vi "Process.vi"(9 "process sync":refnum<notifier>, 10 "TopLevel":refnum<class "TopLevel.lvclass">, 11 "Database in":refnum<class "Database.lvclass">) -> ()   [LabVIEW 2022 SP3, in "Database.lvclass"]
doc: "Developed by Kevin Thompson\nkevin@thompsonengineering.net\n\nCopyright 2018\nThompson Engineering, LLC"
uses:
  Database.lvclass
  DataTypes/Read Data--cluster.ctl
  TopLevel/TopLevel.lvclass
  DataTypes/Process - AppData--cluster.ctl
  DataTypes/Settings--cluster.ctl
  DataTypes/Dependency--cluster.ctl
  DataTypes/Public Events--cluster.ctl
  Common/Controls/TD Async CmdMsg EventData--cluster.ctl
  Common/Controls/TD Sync API Event Data.ctl
  Common/Controls/APIReturnCluster--Cluster.ctl
  Common/Controls/TD Sync API Task State.ctl
  Database.lvclass/Database.ctl
  DataTypes/QuiryBuilderData--Cluster.ctl
  Accessors/Get Settings.vi
  Accessors/Get PublicEvents.vi
  Accessors/Get Dependency.vi
  <vilib>/TELLC/SMQ/Add States to Queue using MultiLine String with vData.vi
panel:
  in  "GetMater":bool
  out "Data":string[][](array[string])
  out "DatabaseReadData":T1
  in  "Exit":bool
  # "local data monitoring"
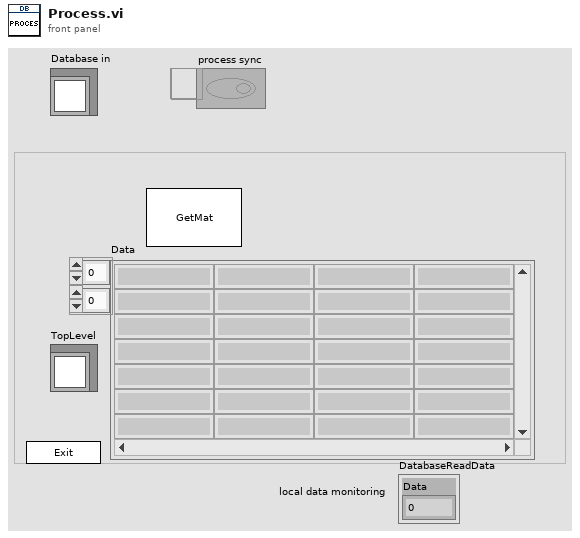
[diagram p1: front panel]
types:
  T1 = typedef "Database.lvclass/Read Data--cluster.ctl" = cluster{"Data":dbl}
  T2 = typedef "Database.lvclass/Process - AppData--cluster.ctl" = cluster{"Core":cluster{"Current VI Reference":refnum<vi>, "Close Panel on Exit?":bool}, "SMQ":refnum<queue>, "Initialized?":bool, "Self Reference":refnum<class "Database.lvclass">, "Simulation?":bool, "process sync":refnum<notifier>, "vData":variant, "Settings":T3, "Dependency":T4, "Public Events":T5, "Tasks":T6[], "CuurentSyncTask":T9, "TO":i32, "Task Start ms":u32, "CurrentTaskReturnValue":variant, "DBRef":refnum<k7>}
  T3 = typedef "Database.lvclass/Settings--cluster.ctl" = cluster{"Simulation":bool}
  T4 = typedef "Database.lvclass/Dependency--cluster.ctl" = cluster{"Config":refnum<class>, "ClassRef":refnum<class>}
  T5 = typedef "Database.lvclass/Public Events--cluster.ctl" = cluster{"Temp01.AsyncCmd Event":refnum<user-event>, "Temp01.AsyncMsg Event":refnum<user-event>, "stop process":refnum<user-event>, "API Incoming Event":refnum<user-event>, "API Executed Event":refnum<user-event>, "API Return Event":refnum<user-event>}
  T6 = typedef "TD Sync API Event Data.ctl" = cluster{"Task":T7, "Command":variant, "Return Value":variant}
  T7 = typedef "APIReturnCluster--Cluster.ctl" = cluster{"Time Stamp":timestamp, "Timeout (ms)":u32, "Task State":T8, "Task Error":errorcluster, "Task ID":string, "Type":enum16{"API", "CMD"}}
  T8 = typedef "TD Sync API Task State.ctl" = enum16{"Completed", "Executing", "Errored", "Pending"}
  T9 = typedef "TD Async CmdMsg EventData--cluster.ctl" = cluster{"Time Stamp":timestamp, "CmdMsg":string, "vData":variant}
  T10 = typedef "QuiryBuilderData--Cluster.ctl" = cluster{"Table":string, "Column":string[], "Value":string[], "WhereColumn":string[], "WhereValue":string[], "OrderBy":string[]}
  T11 = enum32{"invalid app kind", "Development System", "Run Time System", "Student Edition", "Embedded LabVIEW", "Evaluation", "Custom"}
  T12 = enum32{"Invalid", "Standard", "Closed", "Hidden", "Minimized", "Maximized"}
  T13 = typedef "Database.lvclass/AsynCmd_Temp01--enum.ctl" = enum16{"DB.DeleteRecord", "DB.UpdateRecord", "DB.InsertRecord", "DB.SelectRecord", "DB.ExecuteSQLCommand", "DB.FindFirstSlot", "DB.GenericSQLQuery"}
  T14 = enum32{"Invalid", "Standard", "Closed", "Hidden", "Minimized", "Maximized"}[]
  T15 = typedef "TopLevel.lvclass/UserEvents.ctl" = cluster{"API Incoming Event":refnum<user-event>, "API Executed Event":refnum<user-event>, "API Return Event":refnum<user-event>, "Exit Event":refnum<user-event>, "StatusChanged":refnum<user-event>, "DLP GUI Config Changed":refnum<user-event>}
  T16 = cluster{"Current VI Reference":refnum<vi>, "Close Panel on Exit?":bool}
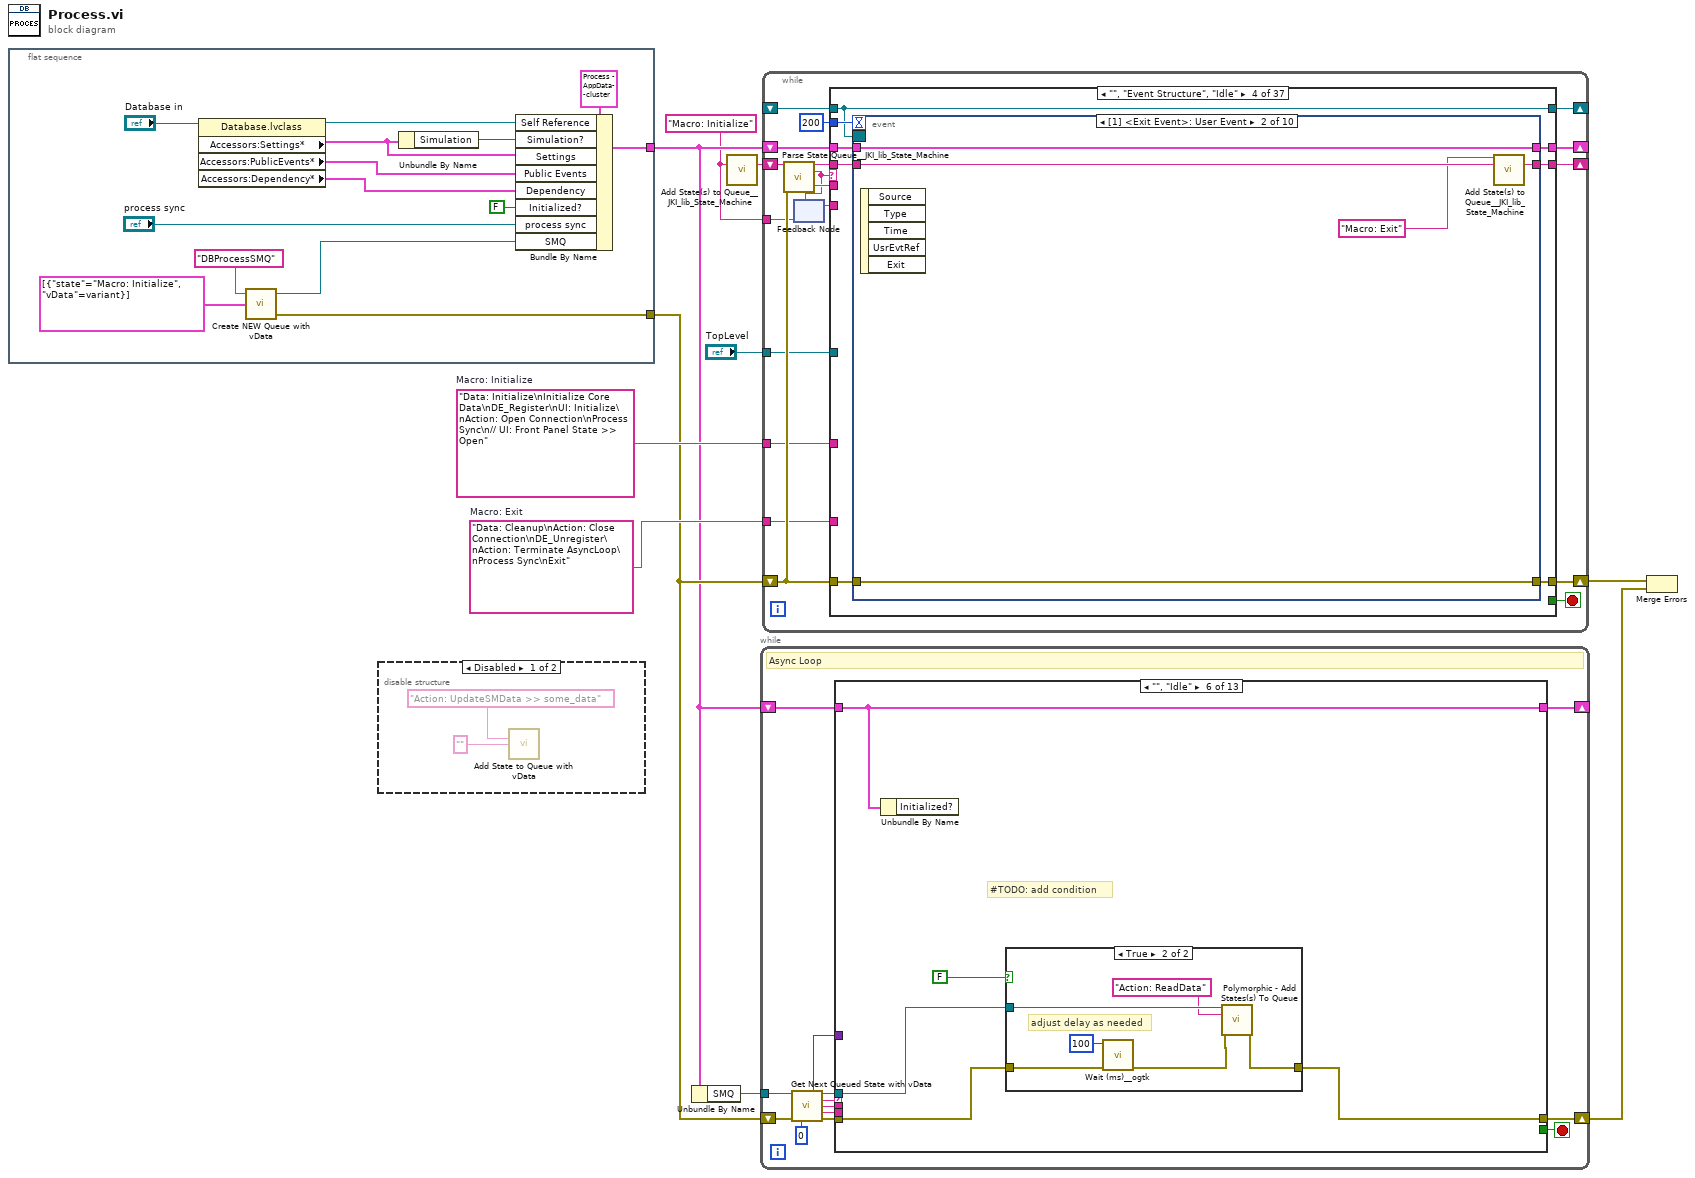
[diagram p0: block diagram]
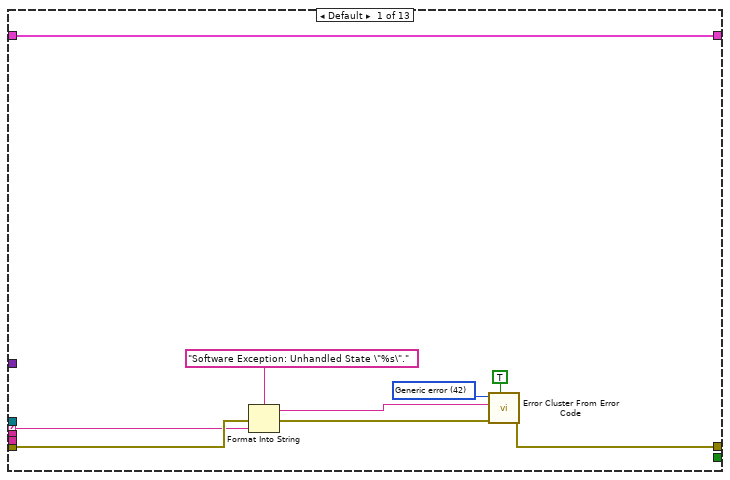
[diagram p3: hidden frame]
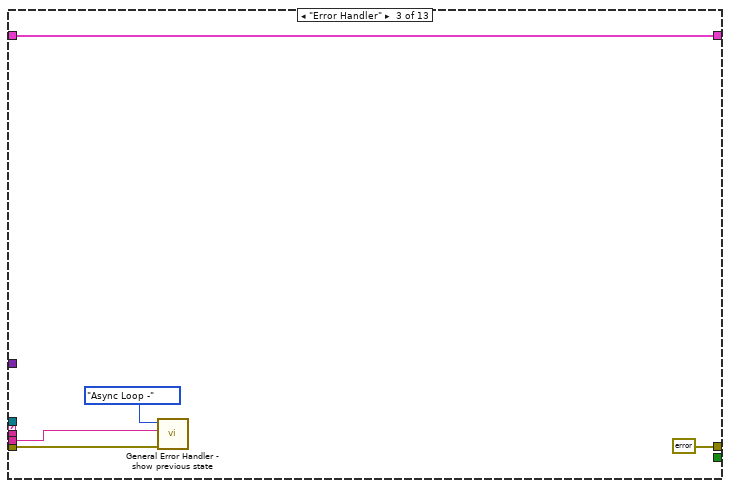
[diagram p5: hidden frame]
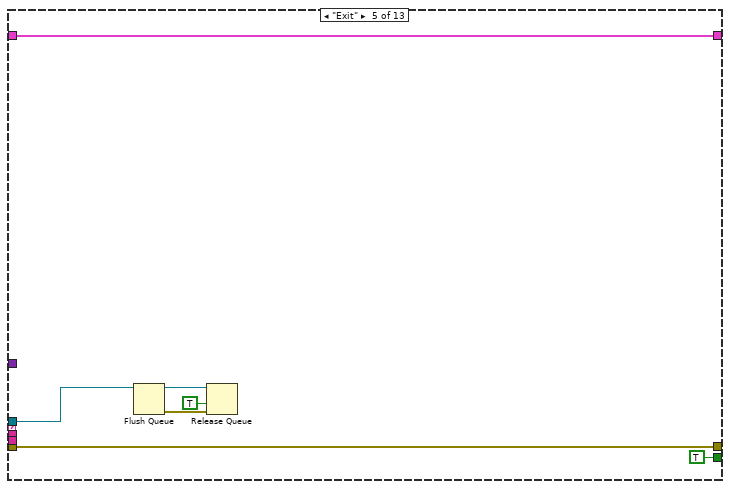
[diagram p7: hidden frame]
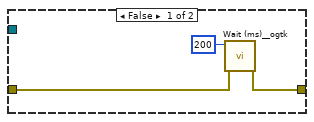
[diagram p8: hidden frame]
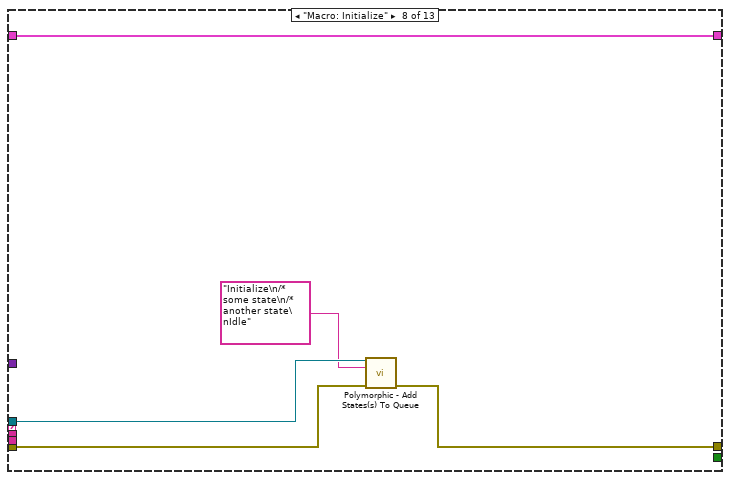
[diagram p10: hidden frame]
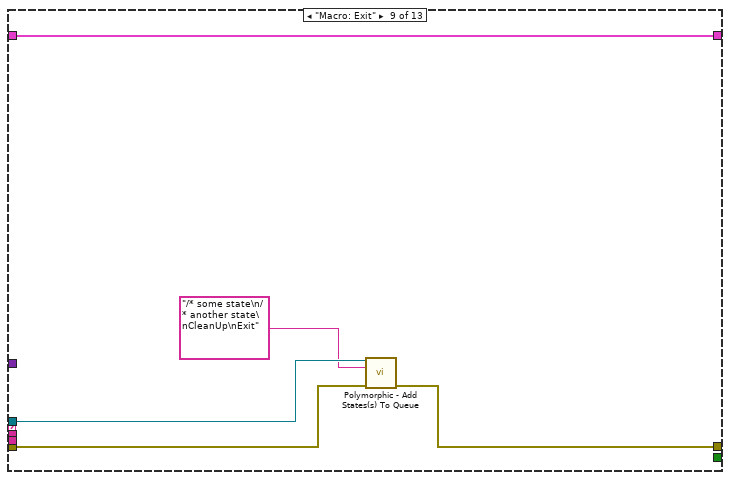
[diagram p11: hidden frame]
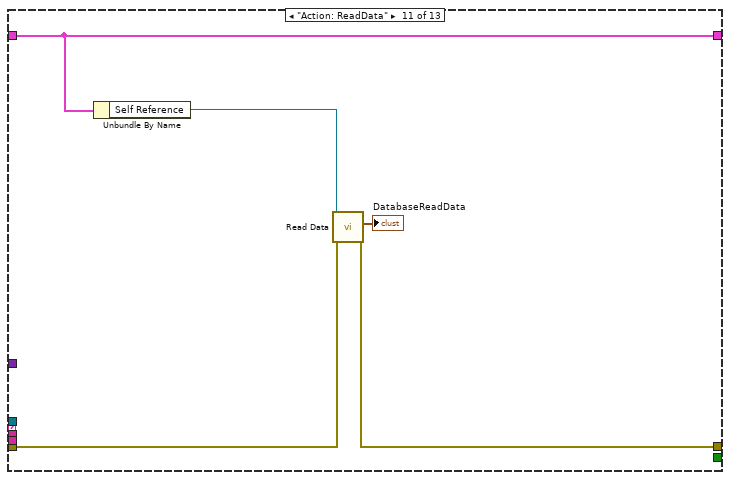
[diagram p13: hidden frame]
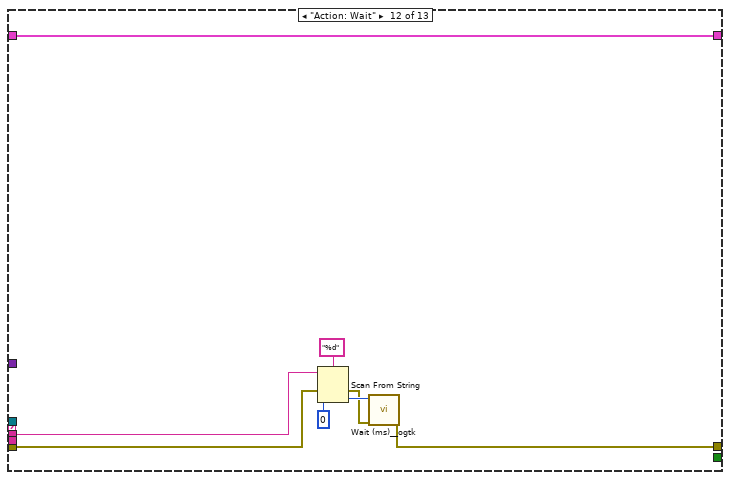
[diagram p14: hidden frame]
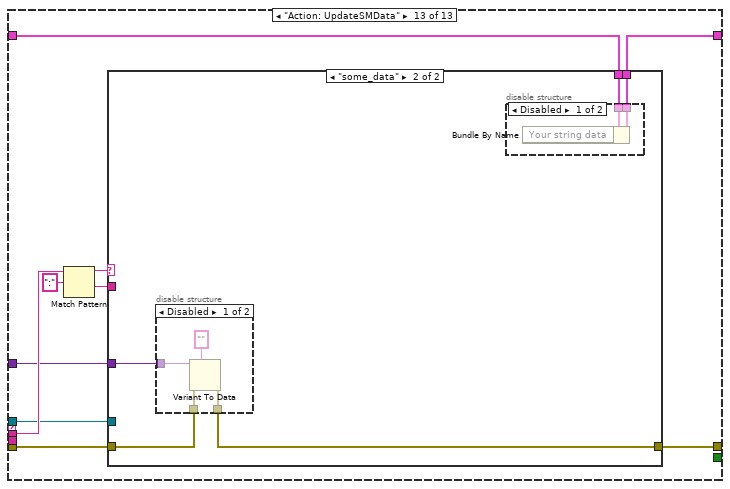
[diagram p15: hidden frame]
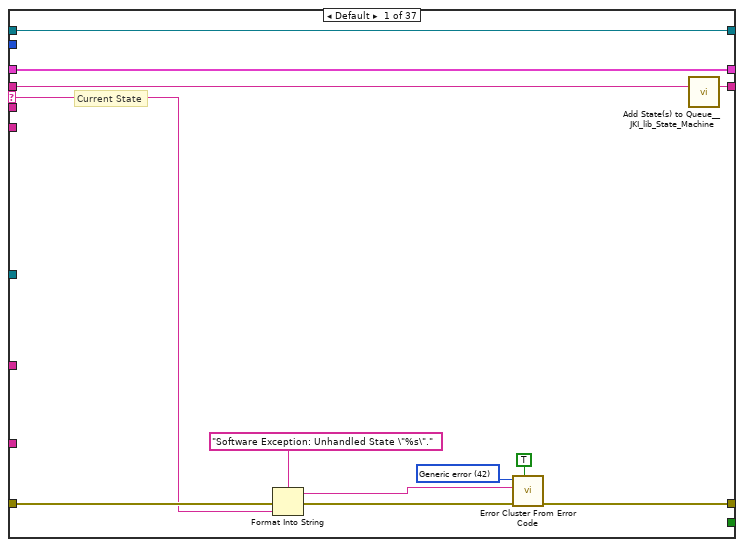
[diagram p19: hidden frame]
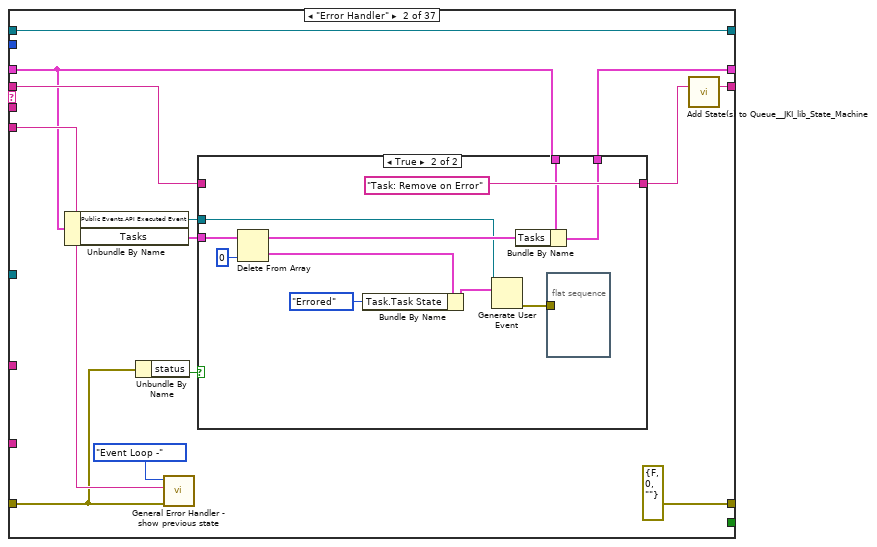
[diagram p20: hidden frame]
diagram:
  w8 = "Data: Cleanup\nAction: Close Connection\nDE_Unregister\nAction: Terminate AsyncLoop\nProcess Sync\nExit"  # Macro: Exit
  w9 = "Data: Initialize\nInitialize Core Data\nDE_Register\nUI: Initialize\nAction: Open Connection\nProcess Sync\n// UI: Front Panel State >> Open"  # Macro: Initialize
  w2 = "Macro: Initialize"
  n1 = flat-sequence {
    tunnel: [w24] -> w5
    tunnel: [w21] -> w7
    frame #0 {
      n2 = property class="Database.lvclass"(reference="Database in") -> (reference out=w17:refnum<class "Database.lvclass">, "Accessors:Settings*"=w12:T3, "Accessors:PublicEvents*"=w14:T5, "Accessors:Dependency*"=w15:T4)  [unwired: 1 in, 1 out]
      n3 = call <vilib>:"Create NEW Queue with vData.vi"("Initial States"=cluster{"state":string, "vData":variant}[] [{"state"="Macro: Initialize", "vData"=variant}], "Name (SMQ)"="DBProcessSMQ") -> ("error out"=w21:errorcluster, "queue out"=w23:refnum<queue>)  [unwired: 2 in]
      n4 = Unbundle By Name(w12) -> ("Simulation"=w13:bool)
      n5 = Bundle By Name(cluster=T2 {"Core"={"Current VI Reference"=refnum, "Close Panel on Exit?"=FALSE}, "SMQ"=refnum, "Initialized?"=FALSE, "Self Reference"=refnum, "Simulation?"=FALSE, "process sync"=refnum, "vData"=variant, "Settings"={"Simulation"=FALSE}, "Dependency"={"Config"=refnum, "ClassRef"=refnum}, "Public Events"={"Temp01.AsyncCmd Event"=refnum, "Temp01.AsyncMsg Event"=refnum, "stop process"=refnum, "API Incoming Event"=refnum, "API Executed Event"=refnum, "API Return Event"=refnum}, "Tasks"=[], "CuurentSyncTask"={"Time Stamp"=timestamp(0 s since 1904-01-01), "CmdMsg"="", "vData"=variant}, "TO"=0, "Task Start ms"=0, "CurrentTaskReturnValue"=variant, "DBRef"=refnum} ("SM2 AppData"), "Self Reference"=w17, "Simulation?"=w13, "Settings"=w12, "Public Events"=w14, "Dependency"=w15, "Initialized?"=FALSE, "process sync"="process sync", "SMQ"=w23) -> (w24:T2)
    }
  }
  n6 = disable-structure shown="Disabled" {
    frame Disabled {
      n7 = call <vilib>:"Add State to Queue with vData.vi"("state in"="Action: UpdateSMData >> some_data", "vData (\"\")"="") -> ()  [unwired: 10 in, 4 out]
    }
    frame Enabled {
    }
  }
  n8 = Unbundle By Name(w5) -> ("SMQ"=w6:refnum<queue>)
  n9 = call <vilib>:"Add State(s) to Queue__JKI_lib_State_Machine.vi"("State(s) in (\"\")"=w2) -> ("States Out"=w10:string)  [unwired: 14 in]
  n10 = while {
    shift-right: [w36] -> w3
    shift-left: w7 -> [w38]
    tunnel: w6 -> [w34]
    shift-right: [w32] -> _
    shift-left: w5 -> [w33]
    stop <- w27 stop-if-true
    # "Async Loop"
    n11 = call <vilib>:"Get Next Queued State with vData.vi"("queue in"=w34, "error in (no error)"=w38, "timeout (100)"=0) -> ("vData out"=w31:variant, "queue out"=w35:refnum<queue>, "Next State"=w39:string, "queued msg"=w29:string, "Prev State"=w28:string, "error out"=w37:errorcluster)  [unwired: 6 in, 1 out]
    n12 = case shown="\"\", \"Idle\"" w39 {
      tunnel: w35 -> [_ _ _ _ w58 w68 _ w84 w89 _ _ _ w111]
      tunnel: w29 -> [_ _ _ _ _ _ _ _ _ _ _ w100 w113]
      selector: w39 -> [w40 _ _ _ _ _ _ _ _ _ _ _ _]
      tunnel: w37 -> [w42 w50 w52 w57 w64 w66 w80 w83 w88 w92 w95 w99 w108]
      tunnel: [w41 w50 errorcluster {"status"=FALSE, "code"=0, "source"=""} ("error constant") w57 w64 w65 w80 w82 w87 w92 w94 w102 w107] -> w36
      tunnel: w33 -> [w48 w49 w55 w56 w63 w67 w79 w85 w90 w91 w97 w105 w110]
      tunnel: [w48 w49 w55 w56 w63 w67 w79 w85 w90 w91 w97 w105 w109] -> w32
      tunnel: w31 -> [_ _ _ _ _ _ _ _ _ _ _ _ w112]
      tunnel: w28 -> [_ _ w51 _ _ _ _ _ _ _ _ _ _]
      tunnel: [_ _ _ _ TRUE _ _ _ _ _ _ _ _] -> w27
      frame Default {
        w44 = 42 items=["No error", "Argument error", "Memory is full", "Out of zone", "End of file", "File already open", "Generic file I/O error", "File not found", "File permission error", "Disk is full", "Duplicate path", "Too many files open", "System feature not enabled", "Resource file not found", "Cannot add resource", "Resource not found", "Image not found", "Image memory error", "Pen does not exist", "Config type invalid", "Config token not found", "Config parse error", "Config memory error", "Bad external code format", "Bad external code offset", "External code not present", "Null window", "Destroy window error", "Null menu", "Print aborted", "Bad print record", "Print driver error", "Windows error during printing", "Memory error during printing", "Print dialog error", "Generic print error", "Invalid device refnum", "Device not found", "Device parameter error", "Device unit error", "Cannot open device", "Device call aborted", "Generic error", "Cancelled by user", "Object ID too low", "Object ID too high", "Object not in heap", "Unknown heap", "Unknown object (invalid DefProc)", "Unknown object (DefProc not in table)", "Message out of range", "Invalid (null) method", "Unknown message", "Manager call not supported", "Bad address", "Network operation in progress", "Network operation timed out", "Connection is busy", "Network attribute not supported", "Network error", "Address in use", "System out of memory", "Connection aborted", "Connection refused", "Not connected", "Already connected", "Connection closed", "Initialization error (interapplication manager)", "Bad occurrence", "Wait on unbound occurrence handler", "Occurrence queue overflow", "Datalog type conflict", "Unused", "Unrecognized type (interapplication manager)", "Memory corrupt", "Failed to make temporary DLL", "Old CIN version", "Drag socket not found", "Failed to load drop-object", "Failed to register OLE object", "Failed to release OLE object", "Format specifier type mismatch", "Unknown format specifier", "Too few format specifiers", "Too many format specifiers", "Scan failed", "Newer CIN version", "Error converting to variant", "Runtime menu error", "Password tampered", "Variant attribute not found", "Incompatible variant data type", "Event data is not available", "Event Store is not present", "Occurrence is not found", "Event Queue is not created", "Event info is not available", "Refnum passed is NULL", "Error retrieving Class GUID", "Error retrieving CoClass GUID", "Error retrieving TypeLib GUID.", "Bad built application magic bytes.", "Specific driver is different from the specific driver associated with the Logical Name.", "There is no session opened to the class driver.", "Max Error", "MAX - Error with config objects", "MAX - Error loading configuration", "MAX - Group not supported"]
        n13 = Format Into String(format string="Software Exception: Unhandled State \"%s\"." ("message"), error in=w42, w40) -> (resulting string=w45:string, error out=w46:errorcluster)  [unwired: 1 in]
        n14 = call <vilib>:"Error Cluster From Error Code.vi"("show call chain? (False)"=TRUE, "error in (no error)"=w46, "error message (\"\")"=w45, "error code (0)"=w44) -> ("error out"=w41:errorcluster)  [unwired: 5 in]
      }
      frame "Initialize" {
      }
      frame "Error Handler" {
        n15 = call "General Error Handler - show previous state.vi"("error in (no error)"=w52, "Previous State"=w51, "Loop Select"=enum16{"Event Loop -", "Async Loop -"}."Async Loop -") -> ()  [unwired: 7 in, 2 out]
      }
      frame "CleanUp" {
      }
      frame "Exit" {
        n16 = Flush Queue(queue=w58) -> (queue out=w61:refnum<queue>, error out=w60:errorcluster)  [unwired: 1 in, 1 out]
        n17 = Release Queue(queue=w61, force destroy? (F)=TRUE, error in (no error)=w60) -> ()  [unwired: 3 out]
      }
      frame "", "Idle" {
        # "#TODO: add condition"
        n18 = Unbundle By Name(w67) -> ()  [unwired: 1 out]
        n19 = case shown="True" FALSE {
          tunnel: w68 -> [_ w78]
          tunnel: w66 -> [w70 w76]
          tunnel: [w71 w73] -> w65
          frame False {
            n20 = call <userlib>:"Wait (ms)__ogtk.vi"("error in (no error)"=w70, "milliseconds to wait"=u32 200) -> ("error out"=w71:errorcluster)  [unwired: 8 in, 1 out]
          }
          frame True {
            # "adjust delay as needed"
            n21 = call <userlib>:"Wait (ms)__ogtk.vi"("error in (no error)"=w76, "milliseconds to wait"=u32 100) -> ("error out"=w75:errorcluster)  [unwired: 8 in, 1 out]
            n22 = call-poly <vilib>:"Polymorphic - Add States(s) To Queue.vi"("queue in"=w78, "state in"="Action: ReadData", "error in"=w75) -> ("error out"=w73:errorcluster)  [unwired: 9 in, 3 out]
          }
        }
      }
      frame "------ Macro ------" {
      }
      frame "Macro: Initialize" {
        n23 = call-poly <vilib>:"Polymorphic - Add States(s) To Queue.vi"("queue in"=w84, "states in"="Initialize\n/* some state\n/* another state\nIdle", "error in"=w83) -> ("error out"=w82:errorcluster)  [unwired: 10 in, 2 out]
      }
      frame "Macro: Exit" {
        n24 = call-poly <vilib>:"Polymorphic - Add States(s) To Queue.vi"("queue in"=w89, "states in"="/* some state\n/* another state\nCleanUp\nExit", "error in"=w88) -> ("error out"=w87:errorcluster)  [unwired: 10 in, 2 out]
      }
      frame "------ Action ------" {
      }
      frame "Action: ReadData" {
        n25 = Unbundle By Name(w97) -> ("Self Reference"=w96:refnum<class "Database.lvclass">)
        n26 = call "Read Data.vi"("error in (no error)"=w95, "Database in"=w96) -> ("error out"=w94:errorcluster, "DatabaseReadData"=→"DatabaseReadData":T1)  [unwired: 7 in, 1 out]
      }
      frame "Action: Wait" {
        n27 = Scan From String(format string="%d", input string=w100, error in=w99, default 1=u32 0) -> (error out=w98:errorcluster, output 1=w104:u32)  [unwired: 1 in, 2 out]
        n28 = call <userlib>:"Wait (ms)__ogtk.vi"("error in (no error)"=w98, "milliseconds to wait"=w104) -> ("error out"=w102:errorcluster)  [unwired: 8 in, 1 out]
      }
      frame "Action: UpdateSMData" {
        n29 = Match Pattern(string=w113, regular expression=":") -> (before substring=w115:string, after substring=w106:string)  [unwired: 1 in, 2 out]
        n30 = case shown="\"some_data\"" w115 {
          tunnel: w112 -> [_ w122]
          tunnel: w111 -> [_ _]
          tunnel: w110 -> [w116 w121]
          tunnel: [w116 w120] -> w109
          tunnel: w108 -> [w117 w119]
          tunnel: [w117 w118] -> w107
          tunnel: w106 -> [_ _]
          frame Default {
            # "#NOTE:\noptionally add error here."
          }
          frame "some_data" {
            n31 = disable-structure shown="Disabled" {
              disable-tunnel: w122 -> [w129 _]
              disable-tunnel: w119 -> [w127 w130]
              disable-tunnel: [w126 w130] -> w118
              frame Disabled {
                n32 = Variant To Data(error in=w127, type="", Variant=w129) -> (error out=w126:errorcluster)  [unwired: 1 out]
              }
              frame Enabled {
              }
            }
            n33 = disable-structure shown="Disabled" {
              disable-tunnel: w121 -> [w124 w125]
              disable-tunnel: [w123 w125] -> w120
              frame Disabled {
                n34 = Bundle By Name(cluster=w124) -> (w123:T2)  [unwired: 1 in]
              }
              frame Enabled {
              }
            }
          }
        }
      }
    }
  }
  n35 = while {
    shift-right: [w142] -> _
    shift-left: w5 -> [w141]
    shift-right: [w145] -> w4
    shift-left: w7 -> [w140]
    shift-right: [w144] -> _
    shift-left: w10 -> [w146]
    shift-right: [w139] -> _
    shift-left: _ -> [w138]
    tunnel: w9 -> [w136]
    tunnel: w8 -> [w135]
    tunnel: w2 -> [w134]
    tunnel: "TopLevel" -> [w131]
    stop <- w143 stop-if-true
    n36 = call <vilib>:"Parse State Queue__JKI_lib_State_Machine.vi"("State Queue"=w146, "Error In (no error)"=w140) -> ("Remaining States"=w148:string, "Current State"=w133:string, "Arguments"=w147:string)  [unwired: 11 in]
    n37 = feedback #1(w134) -> (w132:string)
    n38 = feedback-in #1(w133) -> ()
    n39 = case shown="\"\", \"Event Structure\", \"Idle\"" w133 {
      selector: w133 -> [w150 _ _ _ _ _ _ _ _ _ _ _ _ _ _ _ _ _ _ _ _ _ _ _ _ _ _ _ _ _ _ _ _ _ _ _ _]
      tunnel: w148 -> [w154 w164 w192 w200 w363 w378 w386 w396 w400 w405 w414 w421 w426 w434 w443 w455 w482 w488 w499 w504 w520 w534 w550 w566 w582 w596 w609 w614 w621 w630 w641 w650 w655 w666 w685 w713 w740]
      tunnel: w147 -> [_ _ _ _ _ _ _ _ _ _ _ _ _ _ w438 w449 _ _ _ _ _ _ _ _ _ _ _ _ _ _ w631 _ _ _ _ _ _]
      tunnel: w141 -> [w152 w162 w190 w198 w360 w371 w383 w393 w399 w402 w408 w416 w423 w429 w441 w451 w479 w485 w496 w501 w515 w531 w544 w560 w576 w590 w604 w611 w618 w628 w639 w647 w652 w657 w675 w705 w733]
      tunnel: [w156 errorcluster {"status"=FALSE, "code"=0, "source"=""} ("error out") w189 w197 w361 w375 w379 w394 w397 w403 w412 w417 w424 w430 w439 w452 w480 w486 w497 w502 w513 w529 w542 w558 w574 w588 w601 w612 w616 w623 w632 w642 w653 w661 w678 w704 w732] -> w145
      tunnel: w140 -> [w155 w161 w189 w196 w361 w375 w380 w389 w397 w403 w412 w418 w424 w431 w440 w453 w480 w486 w497 w502 w510 w526 w540 w556 w572 w587 w602 w612 w615 w622 w633 w643 w653 w660 w677 w703 w731]
      tunnel: [w153 w173 w191 w199 w362 w377 w385 w396 w400 w404 w413 w420 w425 w433 w442 w454 w481 w487 w498 w503 w519 w533 w549 w565 w581 w595 w608 w613 w620 w629 w640 w649 w654 w665 w684 w712 w739] -> w144
      tunnel: [_ _ TRUE _ _ _ _ _ _ _ _ _ _ _ _ _ _ _ _ _ _ _ _ _ _ _ _ _ _ _ _ _ _ _ _ _ _] -> w143
      tunnel: [w152 w163 w190 w195 w360 w376 w383 w393 w399 w402 w410 w416 w423 w429 w441 w451 w479 w485 w496 w501 w516 w531 w546 w562 w578 w592 w605 w611 w618 w625 w639 w647 w652 w658 w676 w705 w733] -> w142
      tunnel: [w149 w171 w187 w193 w359 w368 w384 w395 w398 w401 w409 w415 w422 w432 w437 w448 w478 w484 w490 w500 w518 w532 w548 w564 w580 w594 w607 w610 w619 w627 w638 w648 w651 w664 w683 w711 w738] -> w139
      tunnel: w138 -> [w149 w171 w187 w193 w359 w368 w384 _ w398 w401 w409 w415 w422 w432 w437 w448 w478 w484 w490 w500 w518 w532 w548 w564 w580 w594 w607 w610 w619 w627 w638 w648 w651 w664 w683 w711 w738]
      tunnel: 200 ("Timeout") -> [_ _ _ w194 _ _ _ _ _ _ _ _ _ _ _ _ _ _ _ _ _ _ _ _ _ _ _ _ _ _ _ _ _ _ _ _ _]
      tunnel: w136 -> [_ _ _ _ _ _ _ _ _ _ _ _ _ _ _ _ _ w483 _ _ _ _ _ _ _ _ _ _ _ _ _ _ _ _ _ _ _]
      tunnel: w135 -> [_ _ _ _ _ _ _ _ _ _ _ _ _ _ _ _ _ _ w489 _ _ _ _ _ _ _ _ _ _ _ _ _ _ _ _ _ _]
      tunnel: w132 -> [_ w169 _ _ _ _ _ _ _ _ _ _ _ _ _ _ _ _ _ _ _ _ _ _ _ _ _ _ _ _ _ _ _ _ _ _ _]
      tunnel: w131 -> [_ _ _ _ _ _ _ w390 _ _ _ _ _ _ _ _ _ _ _ _ _ _ _ _ _ _ _ _ _ _ _ _ _ _ _ _ _]
      frame Default {
        w159 = 42 items=["No error", "Argument error", "Memory is full", "Out of zone", "End of file", "File already open", "Generic file I/O error", "File not found", "File permission error", "Disk is full", "Duplicate path", "Too many files open", "System feature not enabled", "Resource file not found", "Cannot add resource", "Resource not found", "Image not found", "Image memory error", "Pen does not exist", "Config type invalid", "Config token not found", "Config parse error", "Config memory error", "Bad external code format", "Bad external code offset", "External code not present", "Null window", "Destroy window error", "Null menu", "Print aborted", "Bad print record", "Print driver error", "Windows error during printing", "Memory error during printing", "Print dialog error", "Generic print error", "Invalid device refnum", "Device not found", "Device parameter error", "Device unit error", "Cannot open device", "Device call aborted", "Generic error", "Cancelled by user", "Object ID too low", "Object ID too high", "Object not in heap", "Unknown heap", "Unknown object (invalid DefProc)", "Unknown object (DefProc not in table)", "Message out of range", "Invalid (null) method", "Unknown message", "Manager call not supported", "Bad address", "Network operation in progress", "Network operation timed out", "Connection is busy", "Network attribute not supported", "Network error", "Address in use", "System out of memory", "Connection aborted", "Connection refused", "Not connected", "Already connected", "Connection closed", "Initialization error (interapplication manager)", "Bad occurrence", "Wait on unbound occurrence handler", "Occurrence queue overflow", "Datalog type conflict", "Unused", "Unrecognized type (interapplication manager)", "Memory corrupt", "Failed to make temporary DLL", "Old CIN version", "Drag socket not found", "Failed to load drop-object", "Failed to register OLE object", "Failed to release OLE object", "Format specifier type mismatch", "Unknown format specifier", "Too few format specifiers", "Too many format specifiers", "Scan failed", "Newer CIN version", "Error converting to variant", "Runtime menu error", "Password tampered", "Variant attribute not found", "Incompatible variant data type", "Event data is not available", "Event Store is not present", "Occurrence is not found", "Event Queue is not created", "Event info is not available", "Refnum passed is NULL", "Error retrieving Class GUID", "Error retrieving CoClass GUID", "Error retrieving TypeLib GUID.", "Bad built application magic bytes.", "Specific driver is different from the specific driver associated with the Logical Name.", "There is no session opened to the class driver.", "Max Error", "MAX - Error with config objects", "MAX - Error loading configuration", "MAX - Group not supported"]
        # "Current State"
        n40 = Format Into String(format string="Software Exception: Unhandled State \"%s\"." ("message"), error in=w155, w150) -> (resulting string=w158:string, error out=w157:errorcluster)  [unwired: 1 in]
        n41 = call <vilib>:"Error Cluster From Error Code.vi"("show call chain? (False)"=TRUE, "error in (no error)"=w157, "error message (\"\")"=w158, "error code (0)"=w159) -> ("error out"=w156:errorcluster)  [unwired: 5 in]
        n42 = call <vilib>:"Add State(s) to Queue__JKI_lib_State_Machine.vi"("State(s) in (\"\")"=w154) -> ("States Out"=w153:string)  [unwired: 14 in]
      }
      frame "Error Handler" {
        n43 = Unbundle By Name(w162) -> ("Public Events.API Executed Event"=w168:refnum<user-event>, "Tasks"=w167:T6[])
        n44 = Unbundle By Name(w161) -> ("status"=w166:bool)
        n45 = call "General Error Handler - show previous state.vi"("error in (no error)"=w161, "Previous State"=w169, "Loop Select"=enum16{"Event Loop -", "Async Loop -"}."Event Loop -") -> ()  [unwired: 7 in, 2 out]
        n46 = case shown="True" w166 {
          tunnel: w164 -> [w175 _]
          tunnel: [w175 "Task: Remove on Error"] -> w165
          tunnel: w167 -> [_ w186]
          tunnel: w162 -> [w174 w183]
          tunnel: [w174 w182] -> w163
          tunnel: w168 -> [_ w179]
          frame False {
          }
          frame True {
            n47 = Delete From Array(array=w186, index=0) -> (deleted portion=w178:T6, array with subset deleted=w181:T6[])  [unwired: 1 in]
            n48 = Bundle By Name(cluster=w178, "Task.Task State"=TD_Sync_API_Task_State."Errored") -> (w180:T6)
            n49 = Generate User Event(user event=w179, event data cluster=w180) -> (error out=w176:errorcluster)  [unwired: 2 in, 1 out]
            n50 = Bundle By Name(cluster=w183, "Tasks"=w181) -> (w182:T2)
            n51 = flat-sequence {
              tunnel: w176 -> [_]
              frame #0 {
              }
            }
          }
        }
        n52 = call <vilib>:"Add State(s) to Queue__JKI_lib_State_Machine.vi"("State(s) in (\"\")"=w165) -> ("States Out"=w173:string)  [unwired: 14 in]
      }
      frame "Exit" {
        n53 = call <vilib>:"Add State(s) to Queue__JKI_lib_State_Machine.vi"("State(s) in (\"\")"=w192) -> ("States Out"=w191:string)  [unwired: 14 in]
      }
      frame "", "Event Structure", "Idle" {
        n54 = event shown="[1] <Exit Event>: User Event" {
          selector: w193 -> [_ _ _ _ _ _ _ _ _ _]
          dyn-events: _ -> [_ _ _ _ _ _ _ _ _ _]
          timeout: w194 -> [_ _ _ _ _ _ _ _ _ _]
          tunnel: w200 -> [w204 w209 w220 w237 w293 w313 w319 w322 w329 w345]
          tunnel: [w203 w208 w219 w236 w292 w312 w318 w321 w328 w344] -> w199
          tunnel: w198 -> [w201 w206 w217 w223 w282 w310 w316 w324 w332 w334]
          tunnel: [w202 w207 w218 w221 w268 w311 w317 w325 w333 w342] -> w197
          tunnel: w196 -> [w202 w207 w218 w221 w267 w311 w317 w325 w333 w341]
          tunnel: [w201 w206 w215 w224 w283 w310 w316 w324 w331 w336] -> w195
          event Timeout {
            n55 = event-data() -> ()  [unwired: 1 in, 1 out]
            n56 = call <vilib>:"Add State(s) to Queue__JKI_lib_State_Machine.vi"("State(s) in (\"\")"=w204) -> ("States Out"=w203:string)  [unwired: 14 in]
          }
          event User Event {
            n57 = event-data() -> ()  [unwired: 1 in, 5 out]
            n58 = call <vilib>:"Add State(s) to Queue__JKI_lib_State_Machine.vi"("State(s) in Front (\"\")"="Macro: Exit" ("State(s) in Front (\"\")"), "State(s) in (\"\")"=w209) -> ("States Out"=w208:string)  [unwired: 13 in]
          }
          event "GetMater": Value Change {
            n59 = event-data() -> ()  [unwired: 1 in, 6 out]
            n60 = local write "GetMater"(FALSE ("GetMater")) -> ()
            n61 = Bundle By Name(cluster=T10 {"Table"="", "Column"=[], "Value"=[], "WhereColumn"=[], "WhereValue"=[], "OrderBy"=[]} ("QueryBuilderData"), "Table"="Material", "Column"=string[] ["Material"]) -> (w211:T10)
            n62 = Bundle By Name(cluster=w217, "CuurentSyncTask.vData"=w211) -> (w215:T2)
            n63 = call <vilib>:"Add State(s) to Queue__JKI_lib_State_Machine.vi"("State(s) in Front (\"\")"="Data: GetRecord" ("State(s) in Front (\"\")"), "State(s) in (\"\")"=w220) -> ("States Out"=w219:string)  [unwired: 13 in]
          }
          event User Event {
            n64 = event-data() -> ("Task"=w231:T7, "Command"=w230:variant)  [unwired: 1 in, 5 out]
            n65 = Unbundle By Name(w223) -> ("Tasks"=w226:T6[])
            n66 = Bundle By Name(cluster=T6 {"Task"={"Time Stamp"=timestamp(0 s since 1904-01-01), "Timeout (ms)"=0, "Task State"=enum."Completed", "Task Error"={"status"=FALSE, "code"=0, "source"=""}, "Task ID"="", "Type"=enum."API"}, "Command"=variant, "Return Value"=variant} ("API Event Data"), "Task"=w231, "Command"=w230) -> (w225:T6)
            n67 = Unbundle By Name(w225) -> ("Task.Task ID"=w235:string)
            n68 = String Subset(string=w235, length (rest)=5 ("length (rest)")) -> (substring=w233:string)  [unwired: 1 in]
            n69 = Empty Array?(array=w226) -> (empty?=w227:bool)
            n70 = Equal?(x=w233, y="TopLe") -> (x = y?=w228:bool)
            n71 = case shown="True" w228 {
              tunnel: w227 -> [_ w243]
              tunnel: w226 -> [_ w245]
              tunnel: w225 -> [_ w244]
              tunnel: w223 -> [w238 w242]
              tunnel: [w238 w241] -> w224
              tunnel: [_ w240] -> w222
              tunnel: w221 -> [_ w239]
              frame False {
              }
              frame True {
                n72 = case shown="True" w243 {
                  tunnel: w245 -> [w249 w262]
                  tunnel: w244 -> [w248 w260]
                  tunnel: w242 -> [w247 w258]
                  tunnel: [w246 w257] -> w241
                  tunnel: [_ w253] -> w240
                  tunnel: w239 -> [_ w251]
                  frame False {
                    n73 = Build Array (concatenate)(w249, w248) -> (w250:T6[])
                    n74 = Bundle By Name(cluster=w247, "Tasks"=w250) -> (w246:T2)
                  }
                  frame True {
                    n75 = Unbundle By Name(w260) -> ("Command"=w261:variant)
                    n76 = Build Array (concatenate)(w262, w260) -> (w263:T6[])
                    n77 = Tick Count (ms)() -> (millisecond timer value=w264:u32)
                    n78 = Variant To Data(error in=w251, type=T9 {"Time Stamp"=timestamp(0 s since 1904-01-01), "CmdMsg"="", "vData"=variant} ("Async EvData"), Variant=w261) -> (data=w256:T9, error out=w252:errorcluster)
                    n79 = Unbundle By Name(w256) -> ("CmdMsg"=w254:string)
                    n80 = Bundle By Name(cluster=w258, "TO"=100, "Tasks"=w263, "Task Start ms"=w264, "CuurentSyncTask"=w256) -> (w257:T2)
                    n81 = Format Into String(format string="API: %s", error in=w252, w254) -> (resulting string=w253:string)  [unwired: 1 in, 1 out]
                  }
                }
              }
            }
            n82 = call <vilib>:"Add State(s) to Queue__JKI_lib_State_Machine.vi"("State(s) in Front (\"\")"=w222, "State(s) in (\"\")"=w237) -> ("States Out"=w236:string)  [unwired: 13 in]
          }
          event User Event {
            n83 = event-data() -> ("Task"=w273:T7, "Command"=w287:variant, "Return Value"=w269:variant)  [unwired: 1 in, 4 out]
            n84 = Unbundle By Name(w282) -> ("Public Events.API Return Event"=w270:refnum<user-event>, "Tasks"=w274:T6[])
            n85 = Bundle By Name(cluster=T6 {"Task"={"Time Stamp"=timestamp(0 s since 1904-01-01), "Timeout (ms)"=0, "Task State"=enum."Completed", "Task Error"={"status"=FALSE, "code"=0, "source"=""}, "Task ID"="", "Type"=enum."API"}, "Command"=variant, "Return Value"=variant} ("API Event Data"), "Task"=w273, "Command"=w287, "Return Value"=w269) -> (w284:T6)
            n86 = Delete From Array(array=w274, index=0) -> (deleted portion=w278:T6, array with subset deleted=w272:T6[])  [unwired: 1 in]
            n87 = Unbundle By Name(w284) -> ("Task.Task ID"=w291:string)
            n88 = Unbundle By Name(w278) -> ("Task.Task ID"=w279:string)
            n89 = Unbundle By Name(w273) -> ("Task ID"=w280:string, "Task State"=w271:T8)
            n90 = Empty Array?(array=w274) -> (empty?=w285:bool)
            n91 = String Subset(string=w291, length (rest)=5 ("length (rest)")) -> (substring=w289:string)  [unwired: 1 in]
            n92 = Equal?(x=w279, y=w280) -> (x = y?=w281:bool)
            n93 = Equal?(x=w289, y="TopLe") -> (x = y?=w276:bool)
            n94 = And(x=w281, y=w276) -> (x .and. y?=w275:bool)
            n95 = case shown="True" w275 {
              tunnel: w285 -> [_ _]
              tunnel: w284 -> [_ w296]
              tunnel: w282 -> [w295 w300]
              tunnel: [w295 w299] -> w283
              tunnel: w272 -> [_ w298]
              tunnel: w271 -> [_ w305]
              tunnel: w270 -> [_ w303]
              tunnel: w267 -> [w294 w302]
              tunnel: [w294 w301] -> w268
              tunnel: [_ w297] -> w266
              frame False {
              }
              frame True {
                n96 = Equal?(x=w305, y=TD_Sync_API_Task_State."Errored") -> (x = y?=w308:bool)
                n97 = Select(t="Task: Remove on Error", s=w308, f="Task: Check Pending") -> (s? t:f=w297:string)
                n98 = Bundle By Name(cluster=w300, "Tasks"=w298) -> (w299:T2)
                n99 = Generate User Event(user event=w303, event data cluster=w296, error in=w302) -> (error out=w301:errorcluster)  [unwired: 1 in, 1 out]
              }
            }
            n100 = call <vilib>:"Add State(s) to Queue__JKI_lib_State_Machine.vi"("State(s) in Front (\"\")"=w266, "State(s) in (\"\")"=w293) -> ("States Out"=w292:string)  [unwired: 13 in]
          }
          event "Exit": Value Change {
            n101 = event-data() -> ()  [unwired: 1 in, 1 out]
            n102 = call <vilib>:"Add State(s) to Queue__JKI_lib_State_Machine.vi"("State(s) in Front (\"\")"="Macro: Exit", "State(s) in (\"\")"=w313) -> ("States Out"=w312:string)  [unwired: 13 in]
          }
          event Panel Close? {
            n103 = event-data() -> ()  [unwired: 1 in, 1 out]
            n104 = event-data("Discard?"=TRUE) -> ()  [unwired: 1 in, 1 out]
            n105 = call <vilib>:"Add State(s) to Queue__JKI_lib_State_Machine.vi"("State(s) in Front (\"\")"="Macro: Exit", "State(s) in (\"\")"=w319) -> ("States Out"=w318:string)  [unwired: 13 in]
          }
          event Menu Selection (User) {
            n106 = event-data() -> ("ItemTag"=w323:string)  [unwired: 1 in, 2 out]
            n107 = case shown="\"False\", Default" w323 {
              tunnel: [""] -> w320
              frame "False", Default {
              }
            }
            n108 = call <vilib>:"Add State(s) to Queue__JKI_lib_State_Machine.vi"("State(s) in Front (\"\")"=w320, "State(s) in (\"\")"=w322) -> ("States Out"=w321:string)  [unwired: 13 in]
          }
          event User Event {
            n109 = event-data() -> ("notifier out"=w330:refnum<notifier>)  [unwired: 1 in]
            n110 = Bundle By Name(cluster=w332, "process sync"=w330) -> (w331:T2)
            n111 = call <vilib>:"Add State(s) to Queue__JKI_lib_State_Machine.vi"("State(s) in Front (\"\")"="Macro: Exit", "State(s) in (\"\")"=w329) -> ("States Out"=w328:string)  [unwired: 13 in]
          }
          event User Event {
            n112 = event-data() -> ("CmdMsg"=w339:string, "vData"=w343:variant)  [unwired: 1 in, 1 out]
            n113 = Unbundle By Name(w334) -> ("Self Reference"=w335:refnum<class "Database.lvclass">)
            n114 = call "get async cmd.vi"("error in (no error)"=w341, "Cmd String in"=w339) -> ("error out"=w340:errorcluster, "AsyncCmd"=w338:T13)  [unwired: 8 in]
            n115 = case shown="Default" w338 {
              tunnel: w343 -> [_ w354]
              tunnel: w340 -> [w346 w353]
              tunnel: [w346 w352] -> w342
              tunnel: [_ ""] -> w337
              tunnel: w334 -> [w347 w350]
              tunnel: [w347 w349] -> w336
              tunnel: w335 -> [_ _]
              tunnel: w334 -> [_ _]
              frame Default {
              }
              frame "DB.DeleteRecord" {
                n116 = disable-structure shown="Disabled" {
                  disable-tunnel: w354 -> [w357 _]
                  disable-tunnel: w353 -> [w356 w358]
                  disable-tunnel: [w355 w358] -> w352
                  frame Disabled {
                    n117 = Variant To Data(error in=w356, Variant=w357) -> (error out=w355:errorcluster)  [unwired: 1 in, 1 out]
                  }
                  frame Enabled {
                  }
                }
                n118 = Bundle By Name(cluster=w350, "vData"=variant) -> (w349:T2)
              }
            }
            n119 = call <vilib>:"Add State(s) to Queue__JKI_lib_State_Machine.vi"("State(s) in Front (\"\")"=w337, "State(s) in (\"\")"=w345) -> ("States Out"=w344:string)  [unwired: 13 in]
          }
        }
      }
      frame "---------- Core ----------" {
        n120 = call <vilib>:"Add State(s) to Queue__JKI_lib_State_Machine.vi"("State(s) in (\"\")"=w363) -> ("States Out"=w362:string)  [unwired: 14 in]
      }
      frame "Initialize Core Data" {
        w366 = T14 [enum."Closed", enum."Hidden", enum."Invalid"] items=["Invalid", "Standard", "Closed", "Hidden", "Minimized", "Maximized"]
        # "originally closed?"
        # "exe?"
        n121 = property class="App"() -> ("App.Kind"=w374:T11)  [unwired: 2 in, 2 out]
        n122 = control-ref of="Current VI Reference"() -> (w369:refnum<vi>)
        n123 = property class="VI"() -> ("FP.State"=w367:T12)  [unwired: 2 in, 2 out]
        n124 = Search 1D Array(1D array=w366, element=w367) -> (index of element=w365:i32)  [unwired: 1 in]
        n125 = Equal?(x=w374, y=T11."Run Time System" ("Application:Kind")) -> (x = y?=w372:bool)
        n126 = Greater Than 0?(x=w365) -> (x > 0?=w364:bool)
        n127 = Or(x=w364, y=w372) -> (x .or. y?=w370:bool)
        n128 = Bundle By Name(cluster=w371, "Core.Current VI Reference"=w369, "Core.Close Panel on Exit?"=w370) -> (w376:T2)
        n129 = call <vilib>:"Add State(s) to Queue__JKI_lib_State_Machine.vi"("State(s) in (\"\")"=w378) -> ("States Out"=w377:string)  [unwired: 14 in]
      }
      frame "Process Sync" {
        n130 = Unbundle By Name(w383) -> ("process sync"=w382:refnum<notifier>)
        n131 = Send Notification(notification=TRUE, notifier=w382, error in (no error)=w380) -> (error out=w379:errorcluster)  [unwired: 1 out]
        n132 = call <vilib>:"Add State(s) to Queue__JKI_lib_State_Machine.vi"("State(s) in (\"\")"=w386) -> ("States Out"=w385:string)  [unwired: 14 in]
      }
      frame "DE_Register" {
        n133 = Unbundle By Name(w393) -> ("Public Events"=w392:T5)
        n134 = call-dynamic "GetEvents_TopLevel.vi"("error in (no error)"=w389, "TopLevel in"=w390) -> ("error out"=w388:errorcluster, "UserEvents"=w391:T15)  [unwired: 7 in, 1 out]
        n135 = Unbundle By Name(w391) -> ("Exit Event"=w387:refnum<user-event>)
        n136 = register-events(error in=w388, w392, w387) -> (reference out=w395:refnum<event-registration>, error out=w394:errorcluster)  [unwired: 1 in]
      }
      frame "DE_Unregister" {
        n137 = Unregister For Events(event registration refnum=w398, error in=w397) -> ()  [unwired: 1 out]
      }
      frame "---------- Data ----------" {
        n138 = call <vilib>:"Add State(s) to Queue__JKI_lib_State_Machine.vi"("State(s) in (\"\")"=w405) -> ("States Out"=w404:string)  [unwired: 14 in]
      }
      frame "Data: Initialize" {
        w406 = refnum<k7> refnum  # DBRef
        w407 = T6[] []  # Tasks
        w411 = T16 {"Current VI Reference"=refnum, "Close Panel on Exit?"=FALSE}  # Core
        n139 = Unbundle By Name(w408) -> ()  [unwired: 1 out]
        n140 = Bundle By Name(cluster=w408, "Core"=w411, "Tasks"=w407, "DBRef"=w406) -> (w410:T2)
        n141 = call <vilib>:"Add State(s) to Queue__JKI_lib_State_Machine.vi"("State(s) in (\"\")"=w414) -> ("States Out"=w413:string)  [unwired: 14 in]
      }
      frame "Data: Cleanup" {
        n142 = Unbundle By Name(w416) -> ("Core.Current VI Reference"=w419:refnum<vi>)
        n143 = Close Reference(reference=w419, error in (no error)=w418) -> (error out=w417:errorcluster)
        n144 = call <vilib>:"Add State(s) to Queue__JKI_lib_State_Machine.vi"("State(s) in (\"\")"=w421) -> ("States Out"=w420:string)  [unwired: 14 in]
      }
      frame "---------- UI ----------" {
        n145 = call <vilib>:"Add State(s) to Queue__JKI_lib_State_Machine.vi"("State(s) in (\"\")"=w426) -> ("States Out"=w425:string)  [unwired: 14 in]
      }
      frame "UI: Initialize" {
        n146 = Unbundle By Name(w429) -> ("Core.Current VI Reference"=w428:refnum<vi>)
        n147 = call <userlib>:"Fit VI window to Largest Dec__ogtk.vi"("error in (no error)"=w431, "VI Ref (calling VI)"=w428) -> ("error out"=w430:errorcluster, "dup VI Ref"=w427:refnum<vi>)  [unwired: 4 in]
        n148 = disable-structure shown="Disabled" {
          disable-tunnel: w427 -> [w436 _]
          frame Disabled {
            n149 = property class="VI"(reference=w436, "Front Panel.Title"="*VI Title*" ("Front Panel Window:Title")) -> ()  [unwired: 1 in, 2 out]
          }
          frame Enabled {
          }
        }
        n150 = call <vilib>:"Add State(s) to Queue__JKI_lib_State_Machine.vi"("State(s) in (\"\")"=w434) -> ("States Out"=w433:string)  [unwired: 14 in]
      }
      frame "UI: Cursor Set" {
        # "Argument"
        n151 = case shown="\"Idle\", Default" w438 {
          tunnel: w440 -> [w445 w447]
          tunnel: [w444 w446] -> w439
          frame "Idle", Default {
            n152 = call <vilib>:"Unset Busy.vi"("error in (no error)"=w445) -> ("error out"=w444:errorcluster)  [unwired: 10 in]
          }
          frame "Busy" {
            n153 = call <vilib>:"Set Busy.vi"("error in (no error)"=w447) -> ("error out"=w446:errorcluster)  [unwired: 9 in, 1 out]
          }
        }
        n154 = call <vilib>:"Add State(s) to Queue__JKI_lib_State_Machine.vi"("State(s) in (\"\")"=w443) -> ("States Out"=w442:string)  [unwired: 14 in]
      }
      frame "UI: Front Panel State" {
        # "Argument"
        n155 = Unbundle By Name(w451) -> ("Core.Current VI Reference"=w450:refnum<vi>)
        n156 = case shown="\"Open\", Default" w449 {
          tunnel: w453 -> [w459 w472]
          tunnel: [w461 w473] -> w452
          tunnel: w450 -> [w460 w470]
          frame "Open", Default {
            n157 = property class="VI"(reference=w460, error in=w459) -> (reference out=w457:refnum<vi>, error out=w458:errorcluster, "FP.State"=w456:T12)
            n158 = case shown="\"Closed\"" w456 {
              tunnel: [w464 w467] -> w461
              tunnel: w458 -> [w463 w467]
              tunnel: w457 -> [w462 _]
              frame "Closed" {
                n159 = invoke class="VI" method="FP.Open"(reference=w462, error in=w463, "Activate"=TRUE, "State"=T12."Standard") -> (error out=w464:errorcluster)  [unwired: 1 in, 4 out]
              }
              frame "Standard", Default {
              }
            }
          }
          frame "Close" {
            n160 = property class="VI"(reference=w470, error in=w472) -> (reference out=w469:refnum<vi>, error out=w471:errorcluster, "FP.State"=w468:T12)
            n161 = case shown="\"Standard\", \"Hidden\"..\"Maximized\", Default" w468 {
              tunnel: [w474 w477] -> w473
              tunnel: w471 -> [w474 w476]
              tunnel: w469 -> [_ w475]
              frame "Invalid", "Closed" {
              }
              frame "Standard", "Hidden".."Maximized", Default {
                n162 = invoke class="VI" method="FP.Close"(reference=w475, error in=w476) -> (error out=w477:errorcluster)  [unwired: 1 in, 2 out]
              }
            }
          }
        }
        n163 = call <vilib>:"Add State(s) to Queue__JKI_lib_State_Machine.vi"("State(s) in (\"\")"=w455) -> ("States Out"=w454:string)  [unwired: 14 in]
      }
      frame "---------- Macro ----------" {
        n164 = call <vilib>:"Add State(s) to Queue__JKI_lib_State_Machine.vi"("State(s) in (\"\")"=w482) -> ("States Out"=w481:string)  [unwired: 14 in]
      }
      frame "Macro: Initialize" {
        n165 = call <vilib>:"Add State(s) to Queue__JKI_lib_State_Machine.vi"("State(s) in Front (\"\")"=w483, "State(s) in (\"\")"=w488) -> ("States Out"=w487:string)  [unwired: 13 in]
      }
      frame "Macro: Exit" {
        n166 = Unbundle By Name(w496) -> ("Core.Close Panel on Exit?"=w495:bool)
        n167 = Select(t="UI: Front Panel State >> Close", s=w495, f="") -> (s? t:f=w492:string)
        n168 = call <vilib>:"Add State(s) to Queue__JKI_lib_State_Machine.vi"("State(s) in (\"\")"=w492, "State(s) at Back (\"\")"=w489) -> ("States Out"=w491:string)  [unwired: 13 in]
        n169 = call <vilib>:"Add State(s) to Queue__JKI_lib_State_Machine.vi"("State(s) in Front (\"\")"=w491, "State(s) in (\"\")"=w499) -> ("States Out"=w498:string)  [unwired: 13 in]
      }
      frame "-------- API -----------" {
        n170 = call <vilib>:"Add State(s) to Queue__JKI_lib_State_Machine.vi"("State(s) in (\"\")"=w504) -> ("States Out"=w503:string)  [unwired: 14 in]
      }
      frame "API: DB.SelectRecord" {
        n171 = Unbundle By Name(w515) -> ("DBRef"=w514:refnum<k7>, "CuurentSyncTask.vData"=w511:variant)
        n172 = Variant To Data(error in=w510, type=T10 {"Table"="", "Column"=[], "Value"=[], "WhereColumn"=[], "WhereValue"=[], "OrderBy"=[]} ("QueryBuilderData"), Variant=w511) -> (data=w507:T10, error out=w509:errorcluster)
        n173 = call "BuildSelectQuery.vi"("error in (no error)"=w509, "QueryBuilderData"=w507) -> ("error out"=w508:errorcluster, "Query"=w506:string)  [unwired: 8 in]
        n174 = call "SQL Select.vi"("Connection In"=w514, "SQL Query"=w506, "Error in (no error)"=w508) -> ("Data"=w505:string[][], "Error out"=w513:errorcluster)  [unwired: 14 in, 1 out]
        n175 = Bundle By Name(cluster=w515, "CurrentTaskReturnValue"=w505) -> (w516:T2)
        n176 = call <vilib>:"Add State(s) to Queue__JKI_lib_State_Machine.vi"("State(s) in Front (\"\")"=" Tasks: Completed" ("State(s) in Front (\"\")"), "State(s) in (\"\")"=w520) -> ("States Out"=w519:string)  [unwired: 13 in]
      }
      frame "Data: GetRecord" {
        n177 = Unbundle By Name(w531) -> ("DBRef"=w530:refnum<k7>, "CuurentSyncTask.vData"=w527:variant)
        n178 = Variant To Data(error in=w526, type=T10 {"Table"="", "Column"=[], "Value"=[], "WhereColumn"=[], "WhereValue"=[], "OrderBy"=[]} ("QueryBuilderData"), Variant=w527) -> (data=w523:T10, error out=w525:errorcluster)
        n179 = call "BuildSelectQuery.vi"("error in (no error)"=w525, "QueryBuilderData"=w523) -> ("error out"=w524:errorcluster, "Query"=w522:string)  [unwired: 8 in]
        n180 = call "SQL Select.vi"("Connection In"=w530, "SQL Query"=w522, "Error in (no error)"=w524) -> ("Data"=→"Data":string[][], "Error out"=w529:errorcluster)  [unwired: 14 in, 1 out]
        n181 = call <vilib>:"Add State(s) to Queue__JKI_lib_State_Machine.vi"("State(s) in (\"\")"=w534) -> ("States Out"=w533:string)  [unwired: 14 in]
      }
      frame "API: DB.UpdateRecord" {
        n182 = Unbundle By Name(w544) -> ("DBRef"=w543:refnum<k7>, "CuurentSyncTask.vData"=w539:variant)
        n183 = Variant To Data(error in=w540, type=T10 {"Table"="", "Column"=[], "Value"=[], "WhereColumn"=[], "WhereValue"=[], "OrderBy"=[]} ("QueryBuilderData"), Variant=w539) -> (data=w538:T10, error out=w537:errorcluster)
        n184 = call "BuildUpdateQuery.vi"("error in (no error)"=w537, "QueryBuilderData"=w538) -> ("error out"=w535:errorcluster, "Query"=w536:string)  [unwired: 8 in]
        n185 = Bundle By Name(cluster=w544, "CurrentTaskReturnValue"=variant) -> (w546:T2)
        n186 = call "SQL Execute.vi"("Connection In"=w543, "SQL Query"=w536, "Error in (no error)"=w535) -> ("Error out"=w542:errorcluster)  [unwired: 15 in, 1 out]
        n187 = call <vilib>:"Add State(s) to Queue__JKI_lib_State_Machine.vi"("State(s) in Front (\"\")"=" Tasks: Completed" ("State(s) in Front (\"\")"), "State(s) in (\"\")"=w550) -> ("States Out"=w549:string)  [unwired: 13 in]
      }
      frame "API: DB.InsertRecord" {
        n188 = Unbundle By Name(w560) -> ("DBRef"=w559:refnum<k7>, "CuurentSyncTask.vData"=w555:variant)
        n189 = Variant To Data(error in=w556, type=T10 {"Table"="", "Column"=[], "Value"=[], "WhereColumn"=[], "WhereValue"=[], "OrderBy"=[]} ("QueryBuilderData"), Variant=w555) -> (data=w554:T10, error out=w553:errorcluster)
        n190 = Bundle By Name(cluster=w560, "CurrentTaskReturnValue"=variant) -> (w562:T2)
        n191 = call "BuildUpdateQuery.vi"("error in (no error)"=w553, "QueryBuilderData"=w554) -> ("error out"=w551:errorcluster, "Query"=w552:string)  [unwired: 8 in]
        n192 = call "SQL Execute.vi"("Connection In"=w559, "SQL Query"=w552, "Error in (no error)"=w551) -> ("Error out"=w558:errorcluster)  [unwired: 15 in, 1 out]
        n193 = call <vilib>:"Add State(s) to Queue__JKI_lib_State_Machine.vi"("State(s) in Front (\"\")"=" Tasks: Completed" ("State(s) in Front (\"\")"), "State(s) in (\"\")"=w566) -> ("States Out"=w565:string)  [unwired: 13 in]
      }
      frame "API: DB.DeleteRecord" {
        n194 = Unbundle By Name(w576) -> ("DBRef"=w575:refnum<k7>, "CuurentSyncTask.vData"=w571:variant)
        n195 = Variant To Data(error in=w572, type=T10 {"Table"="", "Column"=[], "Value"=[], "WhereColumn"=[], "WhereValue"=[], "OrderBy"=[]} ("QueryBuilderData"), Variant=w571) -> (data=w568:T10, error out=w570:errorcluster)
        n196 = Bundle By Name(cluster=w576, "CurrentTaskReturnValue"=variant) -> (w578:T2)
        n197 = call "BuildDeleteQuery.vi"("error in (no error)"=w570, "QueryBuilderData"=w568) -> ("error out"=w569:errorcluster, "Query"=w567:string)  [unwired: 8 in]
        n198 = call "SQL Execute.vi"("Connection In"=w575, "SQL Query"=w567, "Error in (no error)"=w569) -> ("Error out"=w574:errorcluster)  [unwired: 15 in, 1 out]
        n199 = call <vilib>:"Add State(s) to Queue__JKI_lib_State_Machine.vi"("State(s) in Front (\"\")"=" Tasks: Completed" ("State(s) in Front (\"\")"), "State(s) in (\"\")"=w582) -> ("States Out"=w581:string)  [unwired: 13 in]
      }
      frame "API: DB.ExecuteSQLCommand" {
        n200 = Unbundle By Name(w590) -> ("DBRef"=w589:refnum<k7>, "CuurentSyncTask.vData"=w586:variant)
        n201 = Variant To Data(error in=w587, type="", Variant=w586) -> (data=w584:string, error out=w583:errorcluster)
        n202 = Bundle By Name(cluster=w590, "CurrentTaskReturnValue"=variant) -> (w592:T2)
        n203 = call "SQL Execute.vi"("Connection In"=w589, "SQL Query"=w584, "Error in (no error)"=w583) -> ("Error out"=w588:errorcluster)  [unwired: 15 in, 1 out]
        n204 = call <vilib>:"Add State(s) to Queue__JKI_lib_State_Machine.vi"("State(s) in Front (\"\")"=" Tasks: Completed" ("State(s) in Front (\"\")"), "State(s) in (\"\")"=w596) -> ("States Out"=w595:string)  [unwired: 13 in]
      }
      frame "API: DB.FindFirstSlot" {
        w598 = 0 ("index (row)")
        # "NOT USED"
        n205 = Unbundle By Name(w604) -> ("DBRef"=w603:refnum<k7>)  [unwired: 1 out]
        n206 = call "SQL Select.vi"("Connection In"=w603, "SQL Query"="#TODO DB first slot query", "Error in (no error)"=w602) -> ("Data"=w599:string[][], "Error out"=w601:errorcluster)  [unwired: 14 in, 1 out]
        n207 = Index Array(array=w599, index (row)=w598, index (col)=w598) -> (element=w597:string)
        n208 = Bundle By Name(cluster=w604, "CurrentTaskReturnValue"=w597) -> (w605:T2)
        n209 = call <vilib>:"Add State(s) to Queue__JKI_lib_State_Machine.vi"("State(s) in Front (\"\")"=" Tasks: Completed" ("State(s) in Front (\"\")"), "State(s) in (\"\")"=w609) -> ("States Out"=w608:string)  [unwired: 13 in]
      }
      frame "---------- Action ----------" {
        n210 = call <vilib>:"Add State(s) to Queue__JKI_lib_State_Machine.vi"("State(s) in (\"\")"=w614) -> ("States Out"=w613:string)  [unwired: 14 in]
      }
      frame "Action: Close Connection" {
        n211 = Unbundle By Name(w618) -> ("DBRef"=w617:refnum<k7>)
        n212 = call "SQL Close.vi"("Connection In"=w617, "Error in (no error)"=w615) -> ("Error out"=w616:errorcluster)  [unwired: 17 in]
        n213 = call <vilib>:"Add State(s) to Queue__JKI_lib_State_Machine.vi"("State(s) in (\"\")"=w621) -> ("States Out"=w620:string)  [unwired: 14 in]
      }
      frame "Action: Open Connection" {
        n214 = call "SQL Open.vi"("ConnectionString In"="DLP", "Error in (no error)"=w622) -> ("Connection Out"=w624:refnum<k7>, "Error out"=w623:errorcluster)  [unwired: 16 in]
        n215 = Bundle By Name(cluster=w628, "DBRef"=w624) -> (w625:T2)
        n216 = call <vilib>:"Add State(s) to Queue__JKI_lib_State_Machine.vi"("State(s) in (\"\")"=w630) -> ("States Out"=w629:string)  [unwired: 14 in]
      }
      frame "Action: Wait" {
        n217 = Scan From String(format string="%d", input string=w631, error in=w633, default 1=u32 0) -> (error out=w637:errorcluster, output 1=w636:u32)  [unwired: 1 in, 2 out]
        n218 = call <userlib>:"Wait (ms)__ogtk.vi"("error in (no error)"=w637, "milliseconds to wait"=w636) -> ("error out"=w632:errorcluster)  [unwired: 8 in, 1 out]
        n219 = call <vilib>:"Add State(s) to Queue__JKI_lib_State_Machine.vi"("State(s) in (\"\")"=w641) -> ("States Out"=w640:string)  [unwired: 14 in]
      }
      frame "Action: Terminate AsyncLoop" {
        n220 = Unbundle By Name(w647) -> ("SMQ"=w646:refnum<queue>)
        n221 = Flush Queue(queue=w646) -> (queue out=w645:refnum<queue>)  [unwired: 1 in, 2 out]
        n222 = call <vilib>:"Add State to Queue with vData.vi"("queue in"=w645, "state in"="Macro: Exit", "error in"=w643) -> ("error out"=w642:errorcluster)  [unwired: 9 in, 3 out]
        n223 = call <vilib>:"Add State(s) to Queue__JKI_lib_State_Machine.vi"("State(s) in (\"\")"=w650) -> ("States Out"=w649:string)  [unwired: 14 in]
      }
      frame "---------- Tasks -----------" {
        n224 = call <vilib>:"Add State(s) to Queue__JKI_lib_State_Machine.vi"("State(s) in (\"\")"=w655) -> ("States Out"=w654:string)  [unwired: 14 in]
      }
      frame "Task: Remove on Error" {
        n225 = Unbundle By Name(w657) -> ("Public Events.API Return Event"=w663:refnum<user-event>, "Tasks"=w662:T6[])
        n226 = for {
          tunnel: w663 -> [w673]
          tunnel: w662 -> [w672] mode=indexing
          shift-right: [w668] -> w661
          shift-left: w660 -> [w669]
          n227 = Get Date/Time In Seconds() -> (seconds since 1Jan1904=w670:timestamp)
          n228 = Bundle By Name(cluster=w672, "Task.Task State"=TD_Sync_API_Task_State."Errored", "Task.Time Stamp"=w670) -> (w671:T6)
          n229 = Generate User Event(user event=w673, event data cluster=w671, error in=w669) -> (error out=w668:errorcluster)  [unwired: 1 in, 1 out]
        }
        n230 = Bundle By Name(cluster=w657, "TO"=-1, "Tasks"=T6[] []) -> (w658:T2)
        n231 = call <vilib>:"Add State(s) to Queue__JKI_lib_State_Machine.vi"("State(s) in (\"\")"=w666) -> ("States Out"=w665:string)  [unwired: 14 in]
      }
      frame "Task: Check Pending" {
        n232 = Unbundle By Name(w675) -> ("Public Events.API Executed Event"=w681:refnum<user-event>, "Task Start ms"=w680:u32, "Tasks"=w679:T6[])
        n233 = Empty Array?(array=w679) -> (empty?=w682:bool)
        n234 = case shown="False" w682 {
          tunnel: w681 -> [_ _]
          tunnel: w677 -> [w696 w702]
          tunnel: [w694 w702] -> w678
          tunnel: w680 -> [_ _]
          tunnel: w679 -> [w700 _]
          tunnel: [w693 _] -> w674
          tunnel: w675 -> [w692 w701]
          tunnel: [w690 w701] -> w676
          frame False {
            n235 = Index Array(array=w700) -> (element=w698:T6)  [unwired: 1 in]
            n236 = Unbundle By Name(w698) -> ("Command"=w697:variant)
            n237 = Variant To Data(error in=w696, type=T9 {"Time Stamp"=timestamp(0 s since 1904-01-01), "CmdMsg"="", "vData"=variant} ("Async EvData"), Variant=w697) -> (data=w687:T9, error out=w695:errorcluster)
            n238 = Tick Count (ms)() -> (millisecond timer value=w691:u32)
            n239 = Unbundle By Name(w687) -> ("CmdMsg"=w686:string)
            n240 = Bundle By Name(cluster=w692, "TO"=100, "Task Start ms"=w691, "CuurentSyncTask"=w687) -> (w690:T2)
            n241 = Format Into String(format string="API: %s", error in=w695, w686) -> (resulting string=w693:string, error out=w694:errorcluster)  [unwired: 1 in]
          }
          frame True {
          }
        }
        n242 = call <vilib>:"Add State(s) to Queue__JKI_lib_State_Machine.vi"("State(s) in Front (\"\")"=w674, "State(s) in (\"\")"=w685) -> ("States Out"=w684:string)  [unwired: 13 in]
      }
      frame "Tasks: Check Timeout" {
        n243 = Unbundle By Name(w705) -> ("Public Events.API Executed Event"=w709:refnum<user-event>, "Task Start ms"=w706:u32, "Tasks"=w708:T6[])
        n244 = Index Array(array=w708) -> (element=w707:T6)  [unwired: 1 in]
        n245 = Empty Array?(array=w708) -> (empty?=w710:bool)
        n246 = case shown="False" w710 {
          tunnel: w709 -> [w716 _]
          tunnel: w703 -> [w721 w730]
          tunnel: [w717 w730] -> w704
          tunnel: w707 -> [w720 _]
          tunnel: w706 -> [w724 _]
          frame False {
            n247 = Unbundle By Name(w720) -> ("Task.Timeout (ms)"=w722:u32)
            n248 = Tick Count (ms)() -> (millisecond timer value=w715:u32)
            n249 = Subtract(x=w715, y=w724) -> (x-y=w723:u32)
            n250 = Bundle By Name(cluster=w720, "Task.Task State"=TD_Sync_API_Task_State."Errored") -> (w719:T6)
            n251 = Greater Or Equal?(x=w723, y=w722) -> (x >= y?=w718:bool)
            n252 = case shown="True" w718 {
              tunnel: w721 -> [w725 w729]
              tunnel: w719 -> [_ w727]
              tunnel: [w725 w728] -> w717
              tunnel: w716 -> [_ w726]
              frame False {
              }
              frame True {
                n253 = Generate User Event(user event=w726, event data cluster=w727, error in=w729) -> (error out=w728:errorcluster)  [unwired: 1 in, 1 out]
              }
            }
          }
          frame True {
          }
        }
        n254 = call <vilib>:"Add State(s) to Queue__JKI_lib_State_Machine.vi"("State(s) in (\"\")"=w713) -> ("States Out"=w712:string)  [unwired: 14 in]
      }
      frame "Tasks: Completed" {
        n255 = Unbundle By Name(w733) -> ("Public Events.API Executed Event"=w736:refnum<user-event>, "Tasks"=w735:T6[], "CurrentTaskReturnValue"=w734:variant)
        n256 = Empty Array?(array=w735) -> (empty?=w737:bool)
        n257 = case shown="False" w737 {
          tunnel: w736 -> [w746 _]
          tunnel: w735 -> [w747 _]
          tunnel: w731 -> [w745 w748]
          tunnel: [w744 w748] -> w732
          tunnel: w734 -> [w741 _]
          frame False {
            n258 = Index Array(array=w747) -> (element=w743:T6)  [unwired: 1 in]
            n259 = Bundle By Name(cluster=w743, "Return Value"=w741) -> (w742:T6)
            n260 = Generate User Event(user event=w746, event data cluster=w742, error in=w745) -> (error out=w744:errorcluster)  [unwired: 1 in, 1 out]
          }
          frame True {
          }
        }
        n261 = call <vilib>:"Add State(s) to Queue__JKI_lib_State_Machine.vi"("State(s) in (\"\")"=w740) -> ("States Out"=w739:string)  [unwired: 14 in]
      }
    }
  }
  n262 = Merge Errors(w4, w3) -> ()  [unwired: 1 out]
